vi "Get Frequency.vi"(8 "error in (no error)":errorcluster, 11 "Handle in":i32) -> (0 "error out":errorcluster, 2 "Frequency (Hz)":i32, 3 "Handle out":i32)   [LabVIEW 2013, in "Thorlabs_MC2000B.lvlib"]
uses:
  <instrlib>/Thorlabs_MC2000B/Thorlabs_MC2000B.lvlib
  <instrlib>/Thorlabs_MC2000B/Library/MC2000CommandLibWin32.dll
  Program Files/National Instruments/LabVIEW 2011/instr.lib/Thorlabs_MC2000B/Library/MC2000CommandLibWin64.dll
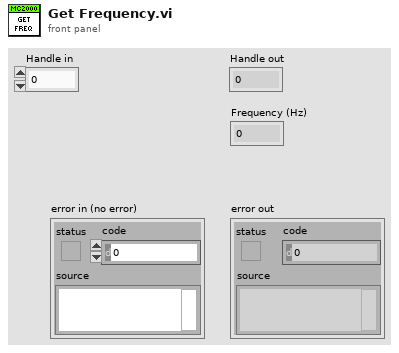
[diagram p1: front panel]
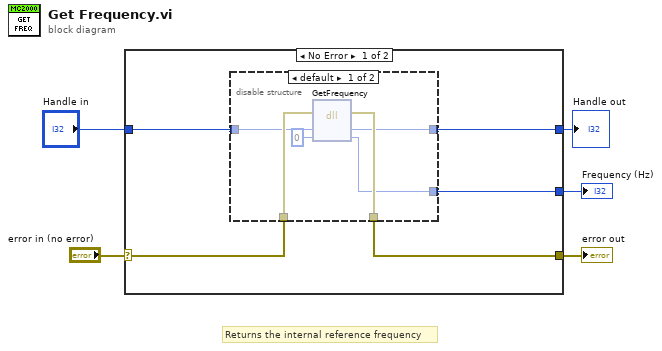
[diagram p0: block diagram]
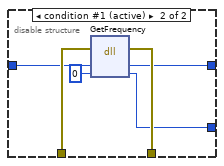
[diagram p2: hidden frame]
diagram:
  # "Returns the internal reference frequency"
  n1 = case shown="No Error" "error in (no error)" {
    selector: "error in (no error)" -> [w10 w24]
    tunnel: [w6 _] -> w5
    tunnel: [w8 w24] -> w4
    tunnel: "Handle in" -> [w9 w23]
    tunnel: [w7 w23] -> w1
    frame No Error {
      n2 = disable-structure shown="default" {
        disable-tunnel: w10 -> [w16 w22]
        disable-tunnel: w9 -> [w15 w21]
        disable-tunnel: [w14 w20] -> w8
        disable-tunnel: [w13 w19] -> w7
        disable-tunnel: [w12 w18] -> w6
        frame condition #0 {
          n3 = dll-call lib="D:/Program Files/National Instruments/LabVIEW 2011/instr.lib/Thorlabs_MC2000B/Library/MC2000CommandLibWin64.dll" fn="GetFrequency"(error in=w16, "handle"=w15, "freq"=0) -> (error out=w14:errorcluster, "handle"=w13:i32, "freq"=w12:i32)  [unwired: 3 in, 1 out]
        }
        frame condition #1 (active) {
          n4 = dll-call lib="C:/Program Files (x86)/National Instruments/LabVIEW 2013/instr.lib/Thorlabs_MC2000B/Library/MC2000CommandLibWin32.dll" fn="GetFrequency"(error in=w22, "handle"=w21, "freq"=0) -> (error out=w20:errorcluster, "handle"=w19:i32, "freq"=w18:i32)  [unwired: 3 in, 1 out]
        }
      }
    }
    frame Error {
    }
  }
  "error out" <- w4
  "Frequency (Hz)" <- w5
  "Handle out" <- w1
